vi "FPGA_IO.vi"() -> ()   [LabVIEW 2017]
uses:
  <vilib>/rvi/Emulation/niFpgaGetClockAttributes.vi
  <vilib>/rvi/Emulation/niFpgaSctlEmulationGetInTimedLoop.vi
  <vilib>/rvi/Emulation/niFpgaEmulationReportErrorSimple.vi
  <vilib>/rvi/eio/common/nirviEmuTemplateMethod_errors.vi
  <vilib>/rvi/Emulation/niFpgaCriticalErrorInLSC.vi
  <vilib>/eio/EIONode/EIONode.xnode
panel:
  in  "x2_read":sgl(slide) scale=-10.0..10.0
  in  "x1_read":sgl(slide) scale=-10.0..10.0
  out "U_read":bool
  in  "stop":bool
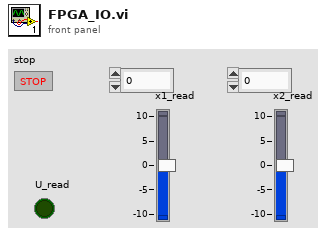
[diagram p1: front panel]
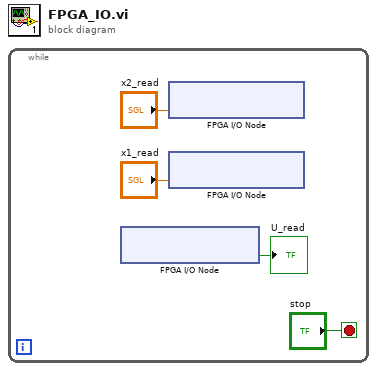
[diagram p0: block diagram]
diagram:
  n1 = while {
    stop <- "stop" stop-if-true
    n2 = xnode "FPGA I/O Node"() -> ("ConnectorA/DIO1"=→"U_read":bool)  [unwired: 1 in, 1 out]
    n3 = xnode "FPGA I/O Node"("ConnectorA/AO1"="x2_read") -> ()  [unwired: 1 in, 1 out]
    n4 = xnode "FPGA I/O Node"("ConnectorA/AO0"="x1_read") -> ()  [unwired: 1 in, 1 out]
  }
